vi "Start motor.vi"(8 "error in":errorcluster, 10 "Motor parameters":T1={"Dirección"=enum."CCW", "Tipo"=enum."Simple", "Velocidad (RPM)"=5.0, "Cantidad de pasos"=1, "Avance (mm)"=0.0}) -> (0 "error out":errorcluster)   [LabVIEW 2020, in "GUI.lvlib"]
doc: "Request to start a motor given is input parameters.\n_____\nCreated using DQMH Event Scripter 6.1.0.128."
uses:
  GUI.lvlib
  Support/Motor parameters.ctl
  Start motor Argument--cluster.ctl
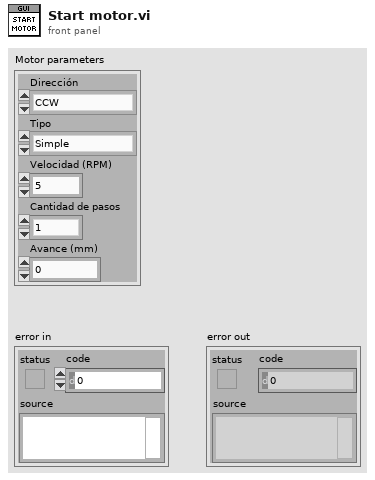
[diagram p1: front panel]
types:
  T1 = typedef "GUI.lvlib/Motor parameters.ctl" = cluster{"Dirección":enum16{"CCW", "CW"}, "Tipo":enum16{"Simple", "Doble"}, "Velocidad (RPM)":dbl, "Cantidad de pasos":i32, "Avance (mm)":dbl}
  T2 = typedef "GUI.lvlib/Start motor Argument--cluster.ctl" = cluster{"Motor params":T1}
  T3 = typedef "GUI.lvlib/Request Events--cluster.ctl" = cluster{"Stop Module":refnum<user-event>, "Show Panel":refnum<user-event>, "Hide Panel":refnum<user-event>, "Get Module Execution Status":refnum<user-event>, "Show Diagram":refnum<user-event>, "Start motor":refnum<user-event>, "Move motor":refnum<user-event>}
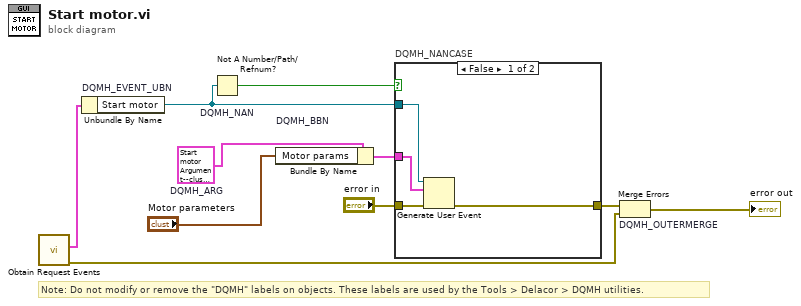
[diagram p0: block diagram]
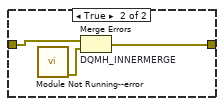
[diagram p2: hidden frame]
diagram:
  w4 = T2 {"Motor params"={"Dirección"=enum."CCW", "Tipo"=enum."Simple", "Velocidad (RPM)"=5.0, "Cantidad de pasos"=1, "Avance (mm)"=0.0}}  # DQMH_ARG
  # "Note: Do not modify or remove the \"DQMH\" labels on objects. These labels are used by the Tools > Delacor > DQMH utilities."
  n1 = call "Obtain Request Events.vi"() -> ("error out"=w2:errorcluster, "GUI Request Events"=w1:T3)  [unwired: 10 in]
  n2 = Unbundle By Name "DQMH_EVENT_UBN"(w1) -> ("Start motor"=w6:refnum<user-event>)
  n3 = Not A Number/Path/Refnum? "DQMH_NAN"(number/path/refnum=w6) -> (NaN/Path/Refnum?=w7:bool)
  n4 = Bundle By Name "DQMH_BBN"(cluster=w4, "Motor params"="Motor parameters") -> (w8:T2)
  n5 = case "DQMH_NANCASE" shown="False" w7 {
    tunnel: "error in" -> [w14 w17]
    tunnel: [w13 w16] -> w5
    tunnel: w6 -> [w12 _]
    tunnel: w8 -> [w11 _]
    frame False {
      n6 = Generate User Event(user event=w12, event data cluster=w11, error in=w14) -> (error out=w13:errorcluster)  [unwired: 1 in, 1 out]
    }
    frame True {
      n7 = call "Module Not Running--error.vi"() -> ("error out"=w15:errorcluster)  [unwired: 11 in]
      n8 = Merge Errors "DQMH_INNERMERGE"(w17, w15) -> (w16:errorcluster)
    }
  }
  n9 = Merge Errors "DQMH_OUTERMERGE"(w5, w2) -> (→"error out":errorcluster)
